vi "Convert C to F.vi"(1 "° C":dbl) -> (0 "° F":dbl)   [LabVIEW 2009]
doc: "Ce VI convertit une mesure en degrés Celsius en degrés Fahrenheit."
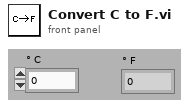
[diagram p1: front panel]
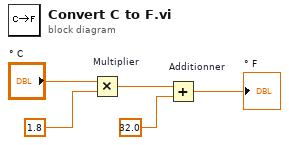
[diagram p0: block diagram]
diagram:
  n1 = Multiply "Multiplier"(x="° C", y=1.8) -> (x*y=w3:dbl)
  n2 = Add "Additionner"(x=w3, y=32.0) -> (x+y=→"° F":dbl)
